vi "Initialize Processes.vi"(8 "Error In":errorcluster, 11 "Dashboard In":refnum<class "Dashboard.lvclass">) -> (0 "Error Out":errorcluster, 3 "Dashboard Out":refnum<class "Dashboard.lvclass">)   [LabVIEW 2019, in "Dashboard.lvclass"]
uses:
  Dashboard.lvclass
  Display Manager/Display Manager.lvclass
  Audio Analyzer/Audio Analyzer.lvclass
  Draw Frame/Draw Frame.lvclass
  Error Handling/Error Handling.lvclass
  Sequencer/Sequencer.lvclass
  Controls/Processes.ctl
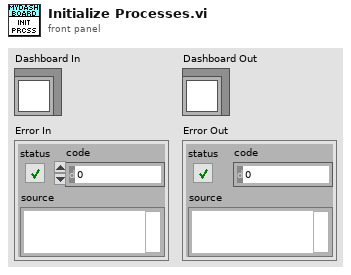
[diagram p1: front panel]
types:
  T1 = typedef "Dashboard.lvclass/Processes.ctl" = cluster{"Display Manager":refnum<class "Display Manager.lvclass">, "Audio Analyzer":refnum<class "Audio Analyzer.lvclass">, "Draw Frame":refnum<class "Draw Frame.lvclass">, "Error Handling":refnum<class "Error Handling.lvclass">, "Sequencer":refnum<class "Sequencer.lvclass">}
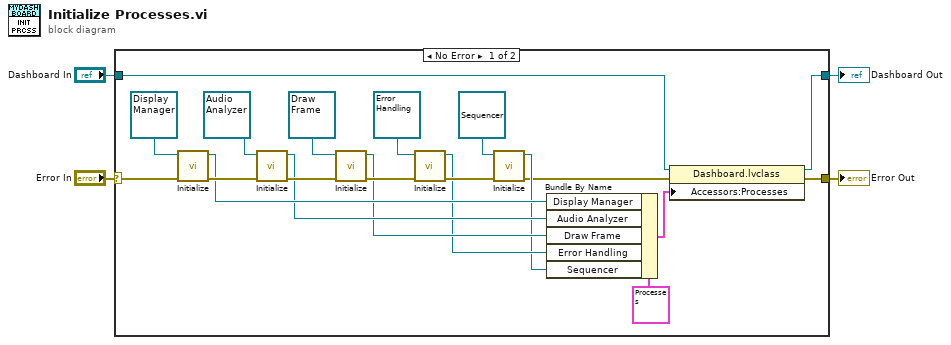
[diagram p0: block diagram]
diagram:
  n1 = case shown="No Error" "Error In" {
    selector: "Error In" -> [w17 w27]
    tunnel: [w25 w27] -> w4
    tunnel: [w24 w26] -> w3
    tunnel: "Dashboard In" -> [w23 w26]
    frame No Error {
      n2 = call-dynamic "Initialize.vi"("Error In"=w17, "Display Manager In"=refnum<class "Display Manager.lvclass"> refnum ("Display Manager")) -> ("Error Out"=w16:errorcluster, "Display Manager Out"=w10:refnum<class "Display Manager.lvclass">)  [unwired: 8 in]
      n3 = call-dynamic "Initialize.vi"("Error In"=w16, "Audio Analyzer In"=refnum<class "Audio Analyzer.lvclass"> refnum ("Audio Analyzer")) -> ("Error Out"=w15:errorcluster, "Audio Analyzer Out"=w9:refnum<class "Audio Analyzer.lvclass">)  [unwired: 8 in]
      n4 = call-dynamic "Initialize.vi"("Error In"=w15, "Draw Frame In"=refnum<class "Draw Frame.lvclass"> refnum ("Draw Frame")) -> ("Error Out"=w14:errorcluster, "Draw Frame Out"=w8:refnum<class "Draw Frame.lvclass">)  [unwired: 8 in]
      n5 = call-dynamic "Initialize.vi"("Error In"=w14, "Error Handling In"=refnum<class "Error Handling.lvclass"> refnum ("Error Handling")) -> ("Error Out"=w13:errorcluster, "Error Handling Out"=w7:refnum<class "Error Handling.lvclass">)  [unwired: 8 in]
      n6 = call-dynamic "Initialize.vi"("Error In"=w13, "Sequencer In"=refnum<class "Sequencer.lvclass"> refnum ("Sequencer")) -> ("Error Out"=w5:errorcluster, "Sequencer Out"=w6:refnum<class "Sequencer.lvclass">)  [unwired: 8 in]
      n7 = Bundle By Name(cluster=T1 {"Display Manager"=refnum, "Audio Analyzer"=refnum, "Draw Frame"=refnum, "Error Handling"=refnum, "Sequencer"=refnum} ("Processes"), "Display Manager"=w10, "Audio Analyzer"=w9, "Draw Frame"=w8, "Error Handling"=w7, "Sequencer"=w6) -> (w21:T1)
      n8 = property class="Dashboard.lvclass"(reference=w23, error in=w5, "Accessors:Processes"=w21) -> (reference out=w24:refnum<class "Dashboard.lvclass">, error out=w25:errorcluster)
    }
    frame Error {
    }
  }
  "Error Out" <- w4
  "Dashboard Out" <- w3
